vi "Clear-object.vi"(8 "error in (no error)":errorcluster, 11 "Object ref in":T1) -> (0 "error out":errorcluster)   [LabVIEW 2013, in "SLMControl.lvlib" / "SC-Main.lvclass"]
uses:
  SC-Main.lvclass
  Object-reference.ctl
  Application-status.ctl
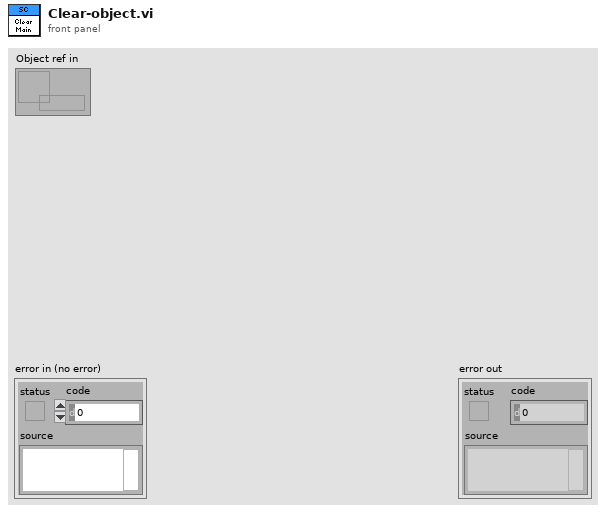
[diagram p1: front panel]
types:
  T1 = typedef "SLMControl.lvlib/SC-Main.lvclass/Object-reference.ctl" = refnum<data-value>
  T2 = typedef "SLMControl.lvlib/SC-Main.lvclass/Application-status.ctl" = enum16{"Idle", "Initialized", "Configured", "Activated", "Started", "Paused", "Stopped", "Reset", "Error", "Exited"}
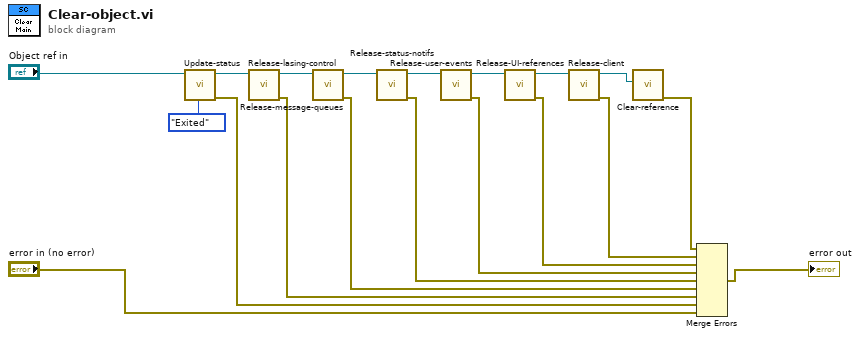
[diagram p0: block diagram]
diagram:
  n1 = call "Update-status.vi"("Status"=Application-status."Exited", "Object ref in"="Object ref in") -> ("error out"=w4:errorcluster, "Object ref out"=w1:T1)  [unwired: 8 in]
  n2 = call "Release-lasing-control.vi"("Main in"=w1) -> ("error out"=w2:errorcluster, "Main out"=w3:T1)  [unwired: 9 in]
  n3 = call "Release-message-queues.vi"("Object ref in"=w3) -> ("error out"=w14:errorcluster, "Object ref out"=w18:T1)  [unwired: 9 in]
  n4 = call "Release-status-notifs.vi"("Object ref in"=w18) -> ("error out"=w13:errorcluster, "Object ref out"=w17:T1)  [unwired: 9 in]
  n5 = call "Release-user-events.vi"("Object ref in"=w17) -> ("error out"=w12:errorcluster, "Object ref out"=w11:T1)  [unwired: 9 in]
  n6 = call "Release-UI-references.vi"("Object ref in"=w11) -> ("error out"=w8:errorcluster, "Object ref out"=w10:T1)  [unwired: 9 in]
  n7 = call "Release-client.vi"("Object ref in"=w10) -> ("error out"=w9:errorcluster, "Object ref out"=w7:T1)  [unwired: 9 in]
  n8 = call "Clear-reference.vi"("Data ref"=w7) -> ("error out"=w16:errorcluster)  [unwired: 10 in]
  n9 = Merge Errors(w16, w9, w8, w12, w13, w14, w2, w4, "error in (no error)") -> (→"error out":errorcluster)
